vi "subject_GetClassAttributes.vi"(1 "return data? (T)":bool=TRUE, 5 "error in (no error)":errorcluster) -> (15 "class attributes ref":T2, 16 "class attributes":T1, 17 "created new?":bool, 19 "error out":errorcluster)   [LabVIEW 2015, in "subject.lvclass"]
doc: "Returns a reference and if wanted the actual data values of the class attributes. This method is used by the subclasses to access parent class attributes."
uses:
  subject.lvclass
  ClassAttributesRef.ctl
  protected/ClassAttributes.ctl
  <vilib>/addons/_AddQ/G#Object/G#Object.lvclass
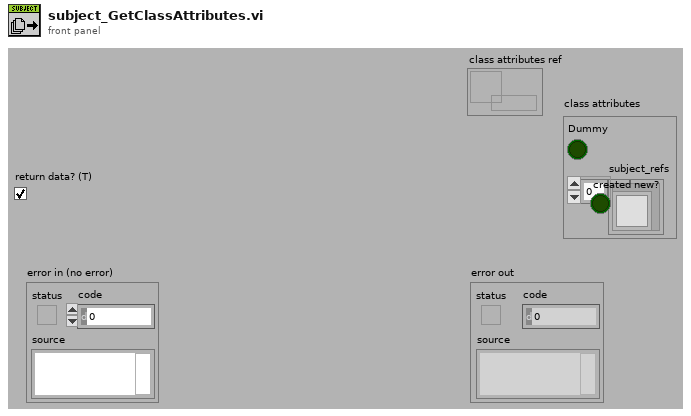
[diagram p1: front panel]
types:
  T1 = typedef "subject.lvclass/ClassAttributes.ctl" = cluster{"Dummy":bool, "subject_refs":refnum<class "subject.lvclass">[]}
  T2 = typedef "subject.lvclass/ClassAttributesRef.ctl" = refnum<data-value>
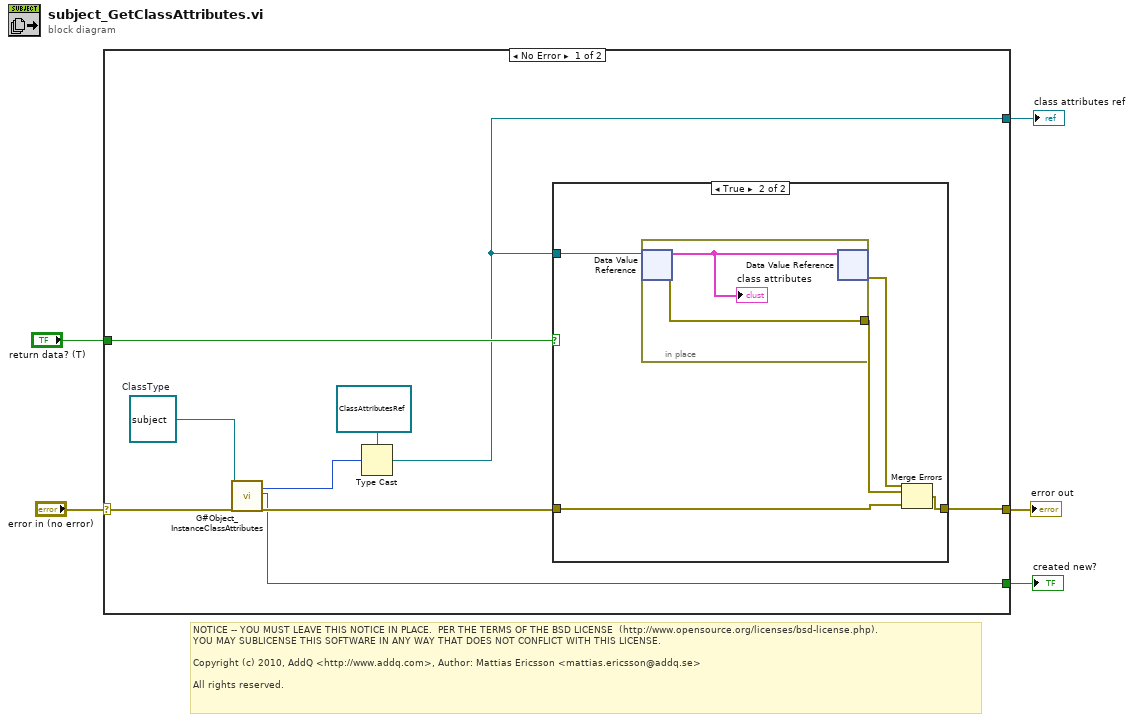
[diagram p0: block diagram]
diagram:
  # "NOTICE -- YOU MUST LEAVE THIS NOTICE IN PLACE.  PER THE TERMS OF THE BSD LICENSE  (http://www.opensource.org/licenses/bsd-license.php).\nYOU MAY SUBLICENSE THIS SOFTWARE IN ANY WAY THAT DOES NOT CONFLICT WITH THIS LICENSE.\n\nCopyright (c) 2010, AddQ <http://www.addq.com>, Author: Mattias Ericsson <mattias.ericsson@addq.se>\n\nAll rights reserved."
  n1 = case shown="No Error" "error in (no error)" {
    selector: "error in (no error)" -> [w10 w23]
    tunnel: [w14 w23] -> w4
    tunnel: [w12 _] -> w2
    tunnel: "return data? (T)" -> [w13 _]
    tunnel: [w6 _] -> w1
    frame No Error {
      w8 = refnum<class "subject.lvclass"> refnum  # ClassType
      n2 = call <vilib>:"G#Object_InstanceClassAttributes.vi"("reference in"=w8, "error in (no error)"=w10) -> ("static attribute ref"=w7:u32, "created new?"=w6:bool, "error out"=w9:errorcluster)  [unwired: 14 in, 1 out]
      n3 = Type Cast(type=T2 refnum ("class attributes ref"), x=w7) -> (*(type *) &x=w12:T2)
      n4 = case shown="True" w13 {
        tunnel: w9 -> [w15 w18]
        tunnel: [w15 w19] -> w14
        tunnel: w12 -> [_ w20]
        frame False {
        }
        frame True {
          n5 = in-place {
            in-place-border: [w22] -> w16
            n6 = in-place-dvr #1(w20) -> (w21:T1, w22:errorcluster)
            "class attributes" <- w21
            n7 = in-place-dvr #1(w21) -> (w17:errorcluster)  [unwired: 1 out]
          }
          n8 = Merge Errors(w17, w16, w18) -> (w19:errorcluster)
        }
      }
    }
    frame Error {
    }
  }
  "error out" <- w4
  "class attributes ref" <- w2
  "created new?" <- w1
